vi "Trajectory.vi"(6 "HomeXY(pixels)":cluster{dbl, dbl}, 7 "PixelmmRatio":dbl format="%#_13g", 8 "Horizontal Edges":T2(array[cluster]) {"Point2 (Real-World)"."Y" format="%.2f"; "Point2 (Real-World)"."X" format="%.2f"; "Point1 (Real-World)"."Y" format="%.2f"; "Point1 (Real-World)"."X" format="%.2f"; "Point2 (Pixels)"."Y" format="%.2f"; "Point2 (Pixels)"."X" format="%.2f"; "Point1 (Pixels)"."Y" format="%.2f"; "Point1 (Pixels)"."X" format="%.2f"}, 9 "Vertical Edges":T2(array[cluster]) {"Point2 (Real-World)"."Y" format="%.2f"; "Point2 (Real-World)"."X" format="%.2f"; "Point1 (Real-World)"."Y" format="%.2f"; "Point1 (Real-World)"."X" format="%.2f"; "Point2 (Pixels)"."Y" format="%.2f"; "Point2 (Pixels)"."X" format="%.2f"; "Point1 (Pixels)"."Y" format="%.2f"; "Point1 (Pixels)"."X" format="%.2f"}, 10 "Puck":T3(array[cluster]) {"Position"."Y" format="%.2f"; "Position"."X" format="%.2f"}, 11 "Players":T3(array[cluster]) {"Position"."Y" format="%.2f"; "Position"."X" format="%.2f"}) -> (0 "Kicker XY":cluster{dbl, dbl}, 1 "ChosenEnergy":dbl, 2 "ChosenPathIdx":i32, 3 "TrajectoryArray":T1, 4 "Angle":dbl, 5 "PuckCentre":cluster{"PuckX":sgl, "PuckY":sgl})   [LabVIEW 2017]
uses:
  <vilib>/imath/engines/lvmath2/RunTimeEngine/IndexReplace/NIMS V(S)=S.vi
  <instcachedir>/0/NIMS V(S)=S_3F4D177D41884A9C969E5FA0B22E4B28.lvgen/NIMS V(S)=S_3F4D177D41884A9C969E5FA0B22E4B28_000.vi
  <vilib>/imathl/engines/lvmath/Functions/Error Handling/Create Error.vi
  <vilib>/imath/engines/lvmath2/RunTimeEngine/IndexRead/NIMS V(S).vi
  <instcachedir>/0/NIMS V(S)_0488751826AF41519A22953C041130DC.lvgen/NIMS V(S)_0488751826AF41519A22953C041130DC_000.vi
  <instcachedir>/0/NIMS V(S)_0488751826AF41519A22953C041130DC.lvgen/NIMS V(S)_0488751826AF41519A22953C041130DC_004.vi
  <vilib>/imath/engines/lvmath2/RunTimeEngine/ErrorHandling/NIMS_Create Error From Enums.vi
  <instcachedir>/0/NIMS V(S)=S_3F4D177D41884A9C969E5FA0B22E4B28.lvgen/NIMS V(S)=S_3F4D177D41884A9C969E5FA0B22E4B28_003.vi
  <instcachedir>/0/NIMS V(S)=S_3F4D177D41884A9C969E5FA0B22E4B28.lvgen/NIMS V(S)=S_3F4D177D41884A9C969E5FA0B22E4B28_004.vi
  <vilib>/imath/engines/lvmath2/RunTimeEngine/BuiltInFunctions/cos/NIMS_cos(C).vi
  <instcachedir>/0/NIMS_cos(C)_D76AB42705D04DD7AB90183D51B32C21.lvgen/NIMS_cos(C)_D76AB42705D04DD7AB90183D51B32C21_001.vi
  <instcachedir>/0/NIMS V(S)=S_3F4D177D41884A9C969E5FA0B22E4B28.lvgen/NIMS V(S)=S_3F4D177D41884A9C969E5FA0B22E4B28_001.vi
  <instcachedir>/0/NIMS V(S)_0488751826AF41519A22953C041130DC.lvgen/NIMS V(S)_0488751826AF41519A22953C041130DC_003.vi
  <vilib>/imath/engines/lvmath2/RunTimeEngine/BuiltInFunctions/sin/NIMS_sin(C).vi
  <instcachedir>/0/NIMS_sin(C)_3AEF00A0D47841AA8A3F5FC7392BEEFD.lvgen/NIMS_sin(C)_3AEF00A0D47841AA8A3F5FC7392BEEFD_001.vi
  <vilib>/imath/engines/lvmath2/RunTimeEngine/RangeToken/NIMS_Range_R3 - Integer.vi
  <instcachedir>/0/NIMS_Range_R3 - Integer_CAFBFE5A2955410088ACA281A3560A2A.lvgen/NIMS_Range_R3 - Integer_CAFBFE5A2955410088ACA281A3560A2A_000.vi
  <vilib>/imath/engines/lvmath2/RunTimeEngine/CommandStatement/MC_CommandStatement_break.vi
  <vilib>/imath/engines/lvmath2/RunTimeEngine/BuiltInFunctions/abs/NIMS_abs(signed).vi
  <instcachedir>/0/NIMS_abs(signed)_C4FCB8E6058B49B797C7C8D53CA5F6EC.lvgen/NIMS_abs(signed)_C4FCB8E6058B49B797C7C8D53CA5F6EC_002.vi
  <vilib>/imath/engines/lvmath/Functions/Error Handling/MergeErrorsWrapper.vi
  <vilib>/imath/engines/lvmath2/RunTimeEngine/BuiltInFunctions/tan/NIMS_tan(C).vi
  <instcachedir>/0/NIMS_tan(C)_C9020A88DA434792876C9862B5DBE795.lvgen/NIMS_tan(C)_C9020A88DA434792876C9862B5DBE795_001.vi
  <vilib>/imath/engines/lvmath2/RunTimeEngine/ArithmeticOperatorToken/NIMS_ArithmeticOperator_power(S).vi
  <instcachedir>/0/NIMS_ArithmeticOperator_power(S)_86B1D76B77564424912EAFCCCC7488ED.lvgen/NIMS_ArithmeticOperator_power(S)_86B1D76B77564424912EAFCCCC7488ED_010.vi
  <vilib>/imath/engines/lvmath2/RunTimeEngine/NodeEndStatement/NIMS_NodeEndStatement_Output.vi
  <instcachedir>/0/NIMS_NodeEndStatement_Output_53EC0D466D134D7ABD903AC30B43404B.lvgen/NIMS_NodeEndStatement_Output_53EC0D466D134D7ABD903AC30B43404B_008.vi
  <instcachedir>/0/NIMS_NodeEndStatement_Output_53EC0D466D134D7ABD903AC30B43404B.lvgen/NIMS_NodeEndStatement_Output_53EC0D466D134D7ABD903AC30B43404B_010.vi
  <vilib>/imath/engines/lvmath2/RunTimeEngine/ErrorHandling/NIMS_Finalize Error.vi
panel:
  out "Angle Array":dbl[](array[numeric])
  out "Lg":dbl[](array[numeric])
  out "Lw Left":dbl[](array[numeric])
  out "Lw right":dbl[](array[numeric])
  out "Puck":sgl[](array[numeric])
  out "isPossible 2":i32[](array[numeric])
  out "energy":dbl[](array[numeric])
  out "playerPoints":dbl[](array[numeric])
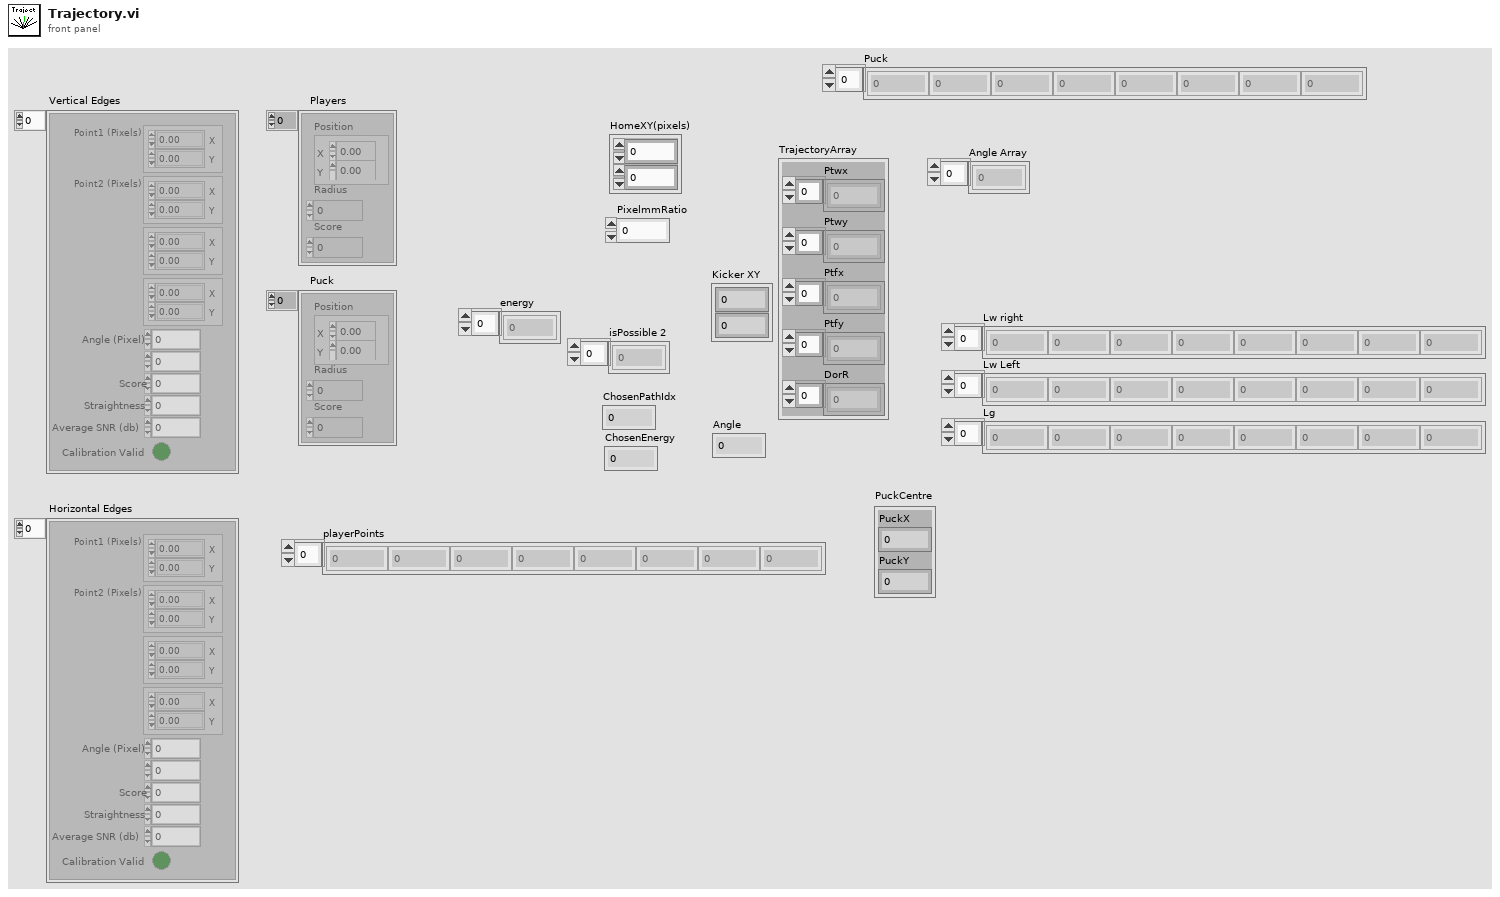
[diagram p1: front panel]
types:
  T1 = cluster{"Ptwx":dbl[], "Ptwy":dbl[], "Ptfx":dbl[], "Ptfy":dbl[], "DorR":i32[]}
  T2 = cluster{"Point1 (Pixels)":cluster{"X":sgl, "Y":sgl}, "Point2 (Pixels)":cluster{"X":sgl, "Y":sgl}, "Point1 (Real-World)":cluster{"X":sgl, "Y":sgl}, "Point2 (Real-World)":cluster{"X":sgl, "Y":sgl}, "Angle (Pixel)":dbl, "Angle (Real-World)":dbl, "Score":dbl, "Straightness":dbl, "Average SNR (db)":dbl, "Calibration Valid":bool}[]
  T3 = cluster{"Position":cluster{"X":sgl, "Y":sgl}, "Radius":dbl, "Score":dbl}[]
  T4 = cluster{"Puck[0]":cluster{"Position":cluster{"X":sgl, "Y":sgl}, "Radius":dbl, "Score":dbl}, "Puck[1]":cluster{"Position":cluster{"X":sgl, "Y":sgl}, "Radius":dbl, "Score":dbl}, "Puck[2]":cluster{"Position":cluster{"X":sgl, "Y":sgl}, "Radius":dbl, "Score":dbl}, "Puck[3]":cluster{"Position":cluster{"X":sgl, "Y":sgl}, "Radius":dbl, "Score":dbl}, "Puck[4]":cluster{"Position":cluster{"X":sgl, "Y":sgl}, "Radius":dbl, "Score":dbl}, "Puck[5]":cluster{"Position":cluster{"X":sgl, "Y":sgl}, "Radius":dbl, "Score":dbl}, "Puck[6]":cluster{"Position":cluster{"X":sgl, "Y":sgl}, "Radius":dbl, "Score":dbl}, "Puck[7]":cluster{"Position":cluster{"X":sgl, "Y":sgl}, "Radius":dbl, "Score":dbl}, "Puck[8]":cluster{"Position":cluster{"X":sgl, "Y":sgl}, "Radius":dbl, "Score":dbl}}
  T5 = cluster{"Position":cluster{"X":sgl, "Y":sgl}, "Radius":dbl, "Score":dbl}
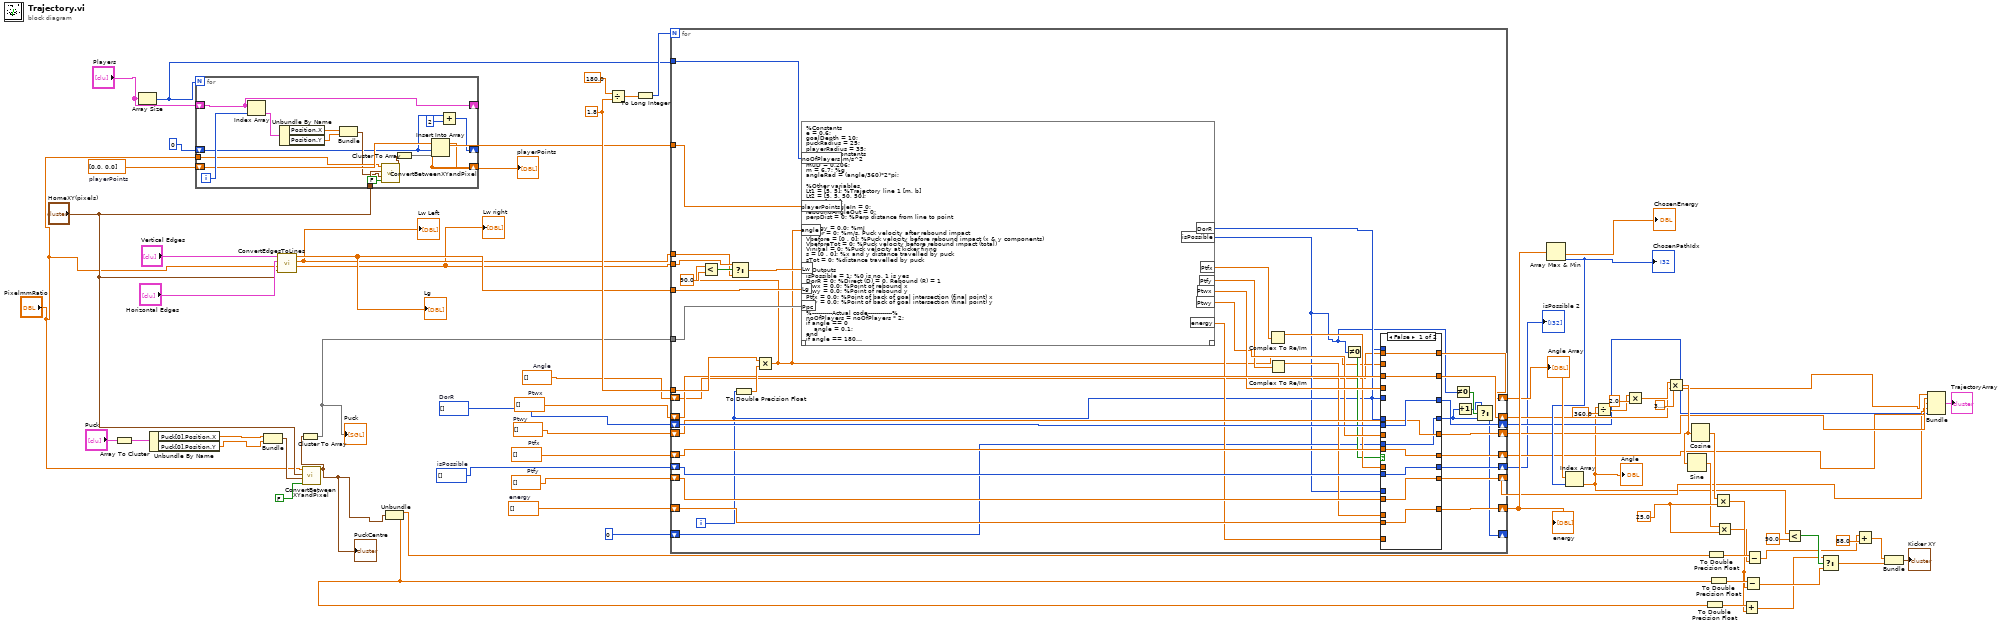
[diagram p0: block diagram]
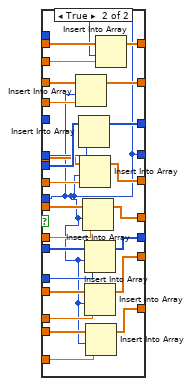
[diagram p2: hidden frame]
diagram:
  w9 = dbl[] []  # Angle
  w35 = i32[] []  # isPossible
  w34 = i32[] []  # DorR
  w36 = dbl[] []  # Ptfy
  w37 = dbl[] []  # Ptwy
  w38 = dbl[] []  # Ptwx
  w49 = 25.0
  w58 = dbl[] []  # energy
  w64 = dbl[] [0.0, 0.0]  # playerPoints
  w66 = dbl[] []  # Ptfx
  w67 = 1.8
  n1 = Array To Cluster(array="Puck") -> (cluster=w61:T4)
  n2 = Array Size(array="Players") -> (size(s)=w39:i32)
  n3 = Unbundle By Name(w61) -> ("Puck[0].Position.X"=w15:sgl, "Puck[0].Position.Y"=w13:sgl)
  n4 = for {
    N: w39 -> [_]
    shift-right: [w82] -> _
    shift-left: "Players" -> [w82]
    shift-right: [w83] -> w63
    shift-left: w64 -> [w84]
    tunnel: "HomeXY(pixels)" -> [w80]
    tunnel: "PixelmmRatio" -> [w78]
    shift-right: [w71] -> _
    shift-left: 0 -> [w73]
    i -> [w85]
    n5 = Index Array(array=w82, index=w85) -> (element=w86:T5)
    n6 = Unbundle By Name(w86) -> ("Position.X"=w77:sgl, "Position.Y"=w76:sgl)
    n7 = Bundle("X"=w77, "Y"=w76) -> (w75:cluster{"X":sgl, "Y":sgl})  [unwired: 1 in]
    n8 = call "ConvertBetweenXYandPixel.vi"("XYtoPixels"=FALSE, "PointToConvert"=w75, "HomeXY(pixels)"=w80, "Pixel/mm"=w78) -> ("Point"=w79:cluster{sgl, sgl})  [unwired: 7 in]
    n9 = Cluster To Array(cluster=w79) -> (array=w81:sgl[])
    n10 = Insert Into Array(array=w84, index=w73, new element=w81) -> (w83:dbl[])
    n11 = Add(x=w73, y=2) -> (x+y=w71:i32)
  }
  "playerPoints" <- w63
  n12 = Bundle("X"=w15, "Y"=w13) -> (w24:cluster{"X":sgl, "Y":sgl})  [unwired: 1 in]
  n13 = call "ConvertEdgesToLines.vi"("HomeXY(pixels)"="HomeXY(pixels)", "PixelmmRatio"="PixelmmRatio", "Horizontal Edges"="Horizontal Edges", "Vertical Edges"="Vertical Edges") -> ("Lw Right"=w16:dbl[], "Lw Left"=w17:dbl[], "Lg"=w18:dbl[])  [unwired: 5 in]
  "Lw right" <- w16
  "Lw Left" <- w17
  "Lg" <- w18
  n14 = call "ConvertBetweenXYandPixel.vi"("XYtoPixels"=FALSE, "PointToConvert"=w24, "HomeXY(pixels)"="HomeXY(pixels)", "Pixel/mm"="PixelmmRatio") -> ("Point"=w8:cluster{sgl, sgl})  [unwired: 7 in]
  "PuckCentre" <- w8
  n15 = Cluster To Array(cluster=w8) -> (array=w19:sgl[])
  "Puck" <- w19
  n16 = Unbundle(w8) -> (w14:sgl, w12:sgl)
  n17 = Divide(x=180.0, y=w67) -> (x/y=w68:dbl)
  n18 = To Long Integer(number=w68) -> (32bit integer=w69:i32)
  n19 = for {
    N: w69 -> [_]
    tunnel: w67 -> [w129]
    shift-right: [w103] -> w29
    shift-left: w66 -> [w118]
    tunnel: w17 -> [w87]
    tunnel: w16 -> [w88]
    tunnel: w18 -> [w127]
    tunnel: w63 -> [w123]
    tunnel: w19 -> [w128]
    shift-right: [w100] -> w57
    shift-left: w58 -> [w115]
    tunnel: w39 -> [w122]
    shift-right: [w106] -> w31
    shift-left: w38 -> [w121]
    shift-right: [w105] -> w27
    shift-left: w34 -> [w120]
    shift-right: [w104] -> w30
    shift-left: w37 -> [w119]
    shift-right: [w102] -> w25
    shift-left: w35 -> [w117]
    shift-right: [w101] -> w28
    shift-left: w36 -> [w116]
    shift-right: [w98] -> w33
    shift-left: w9 -> [w89]
    shift-right: [w90] -> _
    shift-left: 0 -> [w95]
    i -> [w96]
    n20 = To Double Precision Float(number=w96) -> (double precision float=w130:dbl)
    n21 = Multiply(x=w129, y=w130) -> (x*y=w97:dbl)
    n22 = Less?(x=w97, y=90.0) -> (x < y?=w125:bool)
    n23 = Select(t=w88, s=w125, f=w87) -> (s? t:f=w124:dbl[])
    n24 = mathscript code="%Constants\ne = 0.6;\ngoalDepth = 10;\npuckRadius = 25;\nplayerRadius = 35;\n%Energy Constants \ng = 9.81; %m/s^2\nmuD = 0.206;\nm = 6.7; %g\nangleRad = (angle/360)*2*pi;\n\n%Other variables\nLt1 = [5, 5]; %Trajectory line 1 [m, b]\nLt2 = [5, 5, 50, 50];\nPtg = [5, 5];\nreboundAngleIn = 0;\nreboundAngleOut = 0;\nperpDist = 0; %Perp distance from line to point\n\nenergy = 0.0; %mJ\nVafter = 0; %m/s, Puck velocity after rebound impact\nVbefore = [0 , 0]; %Puck velocity before rebound impact (x & y components)\nVbeforeTot = 0; %Puck velocity before rebound impact (total)\nVinitial = 0; %Puck velocity at kicker firing\ns = [0 , 0]; %x and y distance travelled by puck\nsTot = 0; %distance travelled by puck\n\n%Outputs\nisPossible = 1; %0 is no, 1 is yes\nDorR = 0; %Direct (D) = 0, Rebound (R) = 1\nPtwx = 0.0; %Point of rebound x\nPtwy = 0.0; %Point of rebound y\nPtfx = 0.0; %Point of back of goal intersection (final point) x\nPtfy = 0.0; %Point of back of goal intersection (final point) y\n\n%----------Actual code------------%\nnoOfPlayers = noOfPlayers * 2;\nif angle == 0\n    angle = 0.1;\nend\nif angle == 180\n    angle = 179.9;\nend\nif angle == 90\n    Lt1(1) = 0;\n    Lt1(2) = Ppc(2);\nelse\n    Lt1(1) = -1/(tan(angleRad)); % m = tan(theta)\n    Lt1(2) = Ppc(2) - (Lt1(1)*Ppc(1)); % b = y - mx\nend\n\n%offset lines and intersection points\nif angle<90\n    Lw(2) = Lw(2) + (puckRadius/(cos(atan(Lw(1)))));\n    Lw(3) = Lw(3) - puckRadius; %y\n    Lw(4) = Lw(4) + puckRadius;\nelse\n    Lw(2) = Lw(2) - (puckRadius/(cos(atan(Lw(1)))));\n    Lw(3) = Lw(3) - puckRadius;\n    Lw(4) = Lw(4) - puckRadius;\nend\n\nif Lg(1) == 0\n    Lg(2) = Lg(2) - puckRadius;\nelse\n    Lg(2) = Lg(2) - (puckRadius/(sin(atan(Lg(1)))));\nend\nLg(3) = Lg(3) - puckRadius; \nLg(4) = Lg(4) - puckRadius; \nLg(5) = Lg(5) - puckRadius;\nLg(6) = Lg(6) + puckRadius; \n\n%-------------------Intersects with players?----------------%\nfor i = 1:2:noOfPlayers\n    if playerPoints(i) > 0\n        perpDist = ((Lt1(1)*playerPoints(i))+(-1*playerPoints(i+1))+Lt1(2))/(sqrt((Lt1(1)^2)+1));\n        if abs(perpDist) < 30 %(puckRadius+playerRadius)\n            isPossible = 0;\n        end\n    end\nend\n\nif isPossible == 1    \n    %-----------Check if intersects with goal-------------%\n    if Lg(1) == 0\n        Ptg(1) = Lg(2);\n    else\n        Ptg(1) = (Lt1(2)-Lg(2))/(Lg(1)-Lt1(1));\n    end\n    Ptg(2) = (Lt1(1)*Ptg(1))+Lt1(2);\n    if (Ptg(2) < Lg(4)) && (Ptg(2) > Lg(6))\n        if angle == 90\n            Ptfy = Ptg(2);\n        else\n            Ptfy = Ptg(2) + (goalDepth * Lt1(1));\n        end\n        Ptfx = Ptg(1) + goalDepth;\n    elseif ((angle > 90) && (Ptg(2) > Lw(4))) || ((angle < 90) && (Ptg(2) < Lw(4)))\n        DorR = 1;\n        %Check intersection with wall and calculate rebound\n        Ptwx = (Lw(2)-Lt1(2))/(Lt1(1)-Lw(1));\n        Ptwy = (Lw(1)*Ptwx) + Lw(2);\n        %Calculate rebound angle\n        reboundAngleIn = (pi/2) - angleRad;\n       % reboundAngleOut = (pi/2) - (atan(e*tan(reboundAngleIn))); %90 - tan-1(e*tan(angle))\n        reboundAngleOut = (atan(e*tan(reboundAngleIn))); %90 - tan-1(e*tan(angle))\n        %Convert angle and point into line\n        Lt2(1) = 1*tan(reboundAngleOut);\n        Lt2(2) = Ptwy - (Lt2(1)*Ptwx); % b = y - mx\n        %Check intersection with goal\n        if Lg(1) == 0\n            Ptg(1) = Lg(2);\n        else\n            Ptg(1) = (Lt2(2)-Lg(2))/(Lg(1)-Lt2(1));\n        end\n        Ptg(2) = (Lt2(1)*Ptg(1))+Lt2(2);\n        if (Ptg(2) < Lg(4)) && (Ptg(2) > Lg(6))\n            if angle == 90\n                Ptfy = Ptg(2);\n            else\n                Ptfy = Ptg(2) + (goalDepth * Lt2(1));\n            end\n            Ptfx = Ptg(1) + goalDepth;\n            %-------------------Intersects with players?----------------%\n            for i = 1:2:noOfPlayers\n                if playerPoints(i) > 0\n                    perpDist = ((Lt2(1)*playerPoints(i))+(-1*playerPoints(i+1))+Lt2(2))/(sqrt((Lt2(1)^2)+1));\n                    if abs(perpDist) < 40 %(puckRadius+playerRadius)\n                        isPossible = 0;\n                    end\n                end\n            end\n        else\n            isPossible = 0;\n        end\n    else\n        isPossible = 0;\n    end\nend\n\n%need to calculate energy resolution\nif isPossible==1\n    if DorR == 0 %For direct shots\n        s(1) = (Ptfx - Ppc(1)) / 1000; %Find x distance travelled\n        s(2) = (Ptfy - Ppc(2)) / 1000; %Find y distance travelled\n        sTot = SQRT((s(1)^2)+(s(2)^2)); %Find total distance travelled\n        Vinitial = SQRT(2*muD*g*sTot); %Find puck output V required\n        energy = 0.5*m*(Vinitial^2);\n    end\n    if DorR == 1 %For rebound shots\n        s(1) = (Ptfx- Ptwx) / 1000; %Find x distance travelled rebound to final\n        s(2) = (Ptfy - Ptwy) / 1000; %Find y distance travelled rebound to final\n        sTot = SQRT((s(1)^2)+(s(2)^2)); %Find total distance travelled rebound to final\n        Vafter = SQRT(2*muD*g*sTot); %V just after rebound\n        Vbefore(1) = (Vafter * sin(reboundAngleOut)) / e; %x-Velocity component before rebound\n        Vbefore(2) = (Vafter * cos(reboundAngleOut)); %y-Velocity component before rebound\n        VbeforeTot = SQRT((Vbefore(1)^2)+(Vbefore(2)^2)); %Velocity before rebound\n        s(1) = (Ptwx - Ppc(1)) / 1000; %Find x distance travelled inital to rebound\n        s(2) = (Ptwy - Ppc(2)) / 1000; %Find y distance travelled inital to rebound\n        sTot = SQRT((s(1)^2)+(s(2)^2)); %Find total distance travelled inital to rebound\n        Vinitial = SQRT((VbeforeTot^2)+(2*muD*g*sTot)); %Find puck output V required\n        energy = 0.5*m*(Vinitial^2);\n    end\nend"("angle"=w97, "playerPoints"=w123, "Lw"=w124, "Lg"=w127, "Ppc"=w128, "noOfPlayers"=w122) -> ("isPossible"=w94:i32, "DorR"=w107:i32, "energy"=w108:cdb, "Ptfx"=w112:cdb, "Ptfy"=w111:cdb, "Ptwx"=w114:cdb, "Ptwy"=w113:cdb)  [unwired: 1 in, 1 out]
    n25 = Complex To Re/Im(x + iy=w112) -> (x=w110:dbl)  [unwired: 1 out]
    n26 = Complex To Re/Im(x + iy=w111) -> (x=w109:dbl)  [unwired: 1 out]
    n27 = Not Equal To 0?(x=w94) -> (x != 0?=w99:bool)
    n28 = case shown="False" w99 {
      tunnel: w121 -> [w139 w164]
      tunnel: w120 -> [w138 w163]
      tunnel: w119 -> [w136 w162]
      tunnel: w118 -> [w135 w161]
      tunnel: w117 -> [w137 w160]
      tunnel: w116 -> [w134 w159]
      tunnel: w115 -> [w133 w158]
      tunnel: w96 -> [_ _]
      tunnel: w114 -> [_ w157]
      tunnel: w113 -> [_ w156]
      tunnel: w110 -> [_ w155]
      tunnel: w109 -> [_ w154]
      tunnel: w108 -> [_ w153]
      tunnel: w107 -> [_ w152]
      tunnel: w94 -> [_ w151]
      tunnel: [w139 w150] -> w106
      tunnel: [w138 w149] -> w105
      tunnel: [w136 w148] -> w104
      tunnel: [w135 w147] -> w103
      tunnel: [w137 w146] -> w102
      tunnel: [w134 w145] -> w101
      tunnel: [w133 w144] -> w100
      tunnel: w89 -> [w132 w143]
      tunnel: [w132 w142] -> w98
      tunnel: w97 -> [_ w141]
      tunnel: w96 -> [_ _]
      tunnel: w95 -> [w131 w140]
      tunnel: [w131 w140] -> w92
      frame False {
      }
      frame True {
        n29 = Insert Into Array(array=w164, index=w140, new element=w157) -> (w150:dbl[])
        n30 = Insert Into Array(array=w163, new element=w152) -> (w149:i32[])  [unwired: 1 in]
        n31 = Insert Into Array(array=w162, index=w140, new element=w156) -> (w148:dbl[])
        n32 = Insert Into Array(array=w161, index=w140, new element=w155) -> (w147:dbl[])
        n33 = Insert Into Array(array=w160, index=w140, new element=w151) -> (w146:i32[])
        n34 = Insert Into Array(array=w159, index=w140, new element=w154) -> (w145:dbl[])
        n35 = Insert Into Array(array=w158, index=w140, new element=w153) -> (w144:dbl[])
        n36 = Insert Into Array(array=w143, index=w140, new element=w141) -> (w142:dbl[])
      }
    }
    n37 = Not Equal To 0?(x=w94) -> (x != 0?=w93:bool)
    n38 = Increment(x=w92) -> (x+1=w91:i32)
    n39 = Select(t=w91, s=w93, f=w92) -> (s? t:f=w90:i32)
  }
  "energy" <- w57
  "isPossible 2" <- w25
  "Angle Array" <- w33
  n40 = Array Max & Min(array=w57) -> (min value=→"ChosenEnergy":dbl, min index (indices)=w32:i32)  [unwired: 2 out]
  "ChosenPathIdx" <- w32
  n41 = Index Array(array=w33, index=w32) -> (element=w10:dbl)
  "Angle" <- w10
  n42 = Divide(x=w10, y=360.0) -> (x/y=w53:dbl)
  n43 = Multiply(x=w53, y=2.0) -> (x*y=w52:dbl)
  n44 = Multiply(x=w52, y=3.141592653589793) -> (x*y=w50:dbl)
  n45 = Sine(x=w50) -> (sin(x)=w47:dbl)
  n46 = Cosine(x=w50) -> (cos(x)=w48:dbl)
  n47 = To Double Precision Float(number=w12) -> (double precision float=w44:dbl)
  n48 = To Double Precision Float(number=w14) -> (double precision float=w46:dbl)
  n49 = To Double Precision Float(number=w12) -> (double precision float=w45:dbl)
  n50 = Multiply(x=w48, y=w49) -> (x*y=w2:dbl)
  n51 = Multiply(x=w47, y=w49) -> (x*y=w1:dbl)
  n52 = Add(x=w44, y=w2) -> (x+y=w6:dbl)
  n53 = Subtract(x=w45, y=w2) -> (x-y=w7:dbl)
  n54 = Subtract(x=w46, y=w1) -> (x-y=w4:dbl)
  n55 = Less?(x=w10, y=90.0) -> (x < y?=w42:bool)
  n56 = Select(t=w6, s=w42, f=w7) -> (s? t:f=w41:dbl)
  n57 = Add(x=w4, y=88.0) -> (x+y=w3:dbl)
  n58 = Bundle(w3, w41) -> (→"Kicker XY":cluster{dbl, dbl})  [unwired: 1 in]
  n59 = Bundle("Ptwx"=w31, "Ptwy"=w30, "Ptfx"=w29, "Ptfy"=w28, "DorR"=w27) -> (→"TrajectoryArray":T1)  [unwired: 1 in]
